vi "MFLI Enable Scope mode.vi"(11 "Lock-in Handle":T1 {"Handle" format="0x%08x"; "Conn" format="0x%08x"}) -> (3 "Handle Out":T1 {"Handle" format="0x%08x"; "Conn" format="0x%08x"})   [LabVIEW 2022 SP3, in "Lock-in module.lvlib"]
uses:
  Lock-in module.lvlib
  <instrlib>/Zurich Instruments LabOne/Public/ziTypeHandle.ctl
  <instrlib>/Zurich Instruments LabOne/Public/Configure/ziSetValueDoubleArray.vi
  <instrlib>/Zurich Instruments LabOne/Zurich Instruments LabOne.lvlib
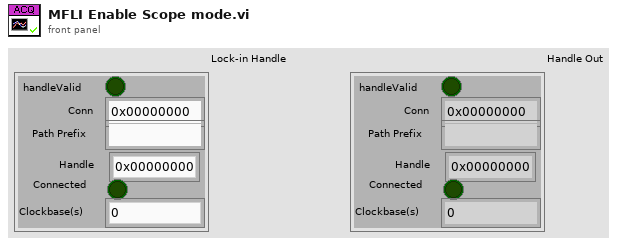
[diagram p1: front panel]
types:
  T1 = typedef "Zurich Instruments LabOne.lvlib/ziTypeHandle.ctl" = cluster{"handleValid":bool, "Conn":u64, "Path Prefix":string, "Handle":u64, "Connected":bool, "Clockbase(s)":dbl}
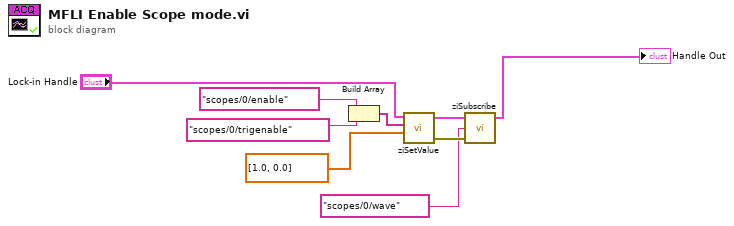
[diagram p0: block diagram]
diagram:
  n1 = Build Array("scopes/0/enable", "scopes/0/trigenable") -> (w3:string[])
  n2 = call-poly <instrlib>:"ziSetValue.vi"("Values"=dbl[] [1.0, 0.0] ("Value"), "Paths"=w3, "Handle In"="Lock-in Handle") -> ("Error Out"=w8:errorcluster, "Handle Out"=w6:T1)  [unwired: 2 in]
  n3 = call <instrlib>:"ziSubscribe.vi"("error in"=w8, "Path ()"="scopes/0/wave" ("Path"), "Handle In"=w6) -> ("Handle Out"=→"Handle Out":T1)  [unwired: 1 in, 1 out]
